vi "select_images.vi"(8 "error in (no error)":errorcluster, 9 "Select":bool, 10 "All":bool, 11 "dict of HIS IN":variant) -> (0 "error out":errorcluster, 3 "dict of HIS OUT":variant)   [LabVIEW 2015]
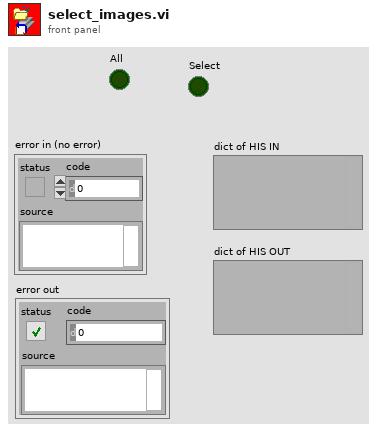
[diagram p1: front panel]
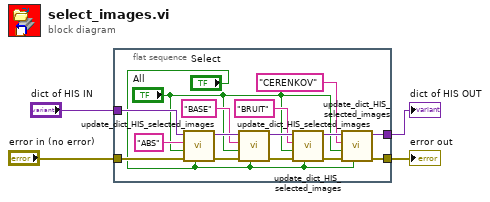
[diagram p0: block diagram]
diagram:
  n1 = flat-sequence {
    tunnel: "dict of HIS IN" -> [w20]
    tunnel: [w16] -> w3
    tunnel: "error in (no error)" -> [w15]
    tunnel: [w11] -> w1
    frame #0 {
      n2 = call "update_dict_HIS_selected_images.vi"("Select"="Select", "error in (no error)"=w15, "All"="All", "type"="ABS" ("name"), "dict of HIS IN"=w20) -> ("error out"=w14:errorcluster, "dict of HIS OUT"=w19:variant)  [unwired: 5 in]
      n3 = call "update_dict_HIS_selected_images.vi"("Select"="Select", "error in (no error)"=w14, "All"="All", "type"="BASE" ("name"), "dict of HIS IN"=w19) -> ("error out"=w13:errorcluster, "dict of HIS OUT"=w18:variant)  [unwired: 5 in]
      n4 = call "update_dict_HIS_selected_images.vi"("Select"="Select", "error in (no error)"=w13, "All"="All", "type"="BRUIT" ("name"), "dict of HIS IN"=w18) -> ("error out"=w12:errorcluster, "dict of HIS OUT"=w17:variant)  [unwired: 5 in]
      n5 = call "update_dict_HIS_selected_images.vi"("Select"="Select", "error in (no error)"=w12, "All"="All", "type"="CERENKOV" ("name"), "dict of HIS IN"=w17) -> ("error out"=w11:errorcluster, "dict of HIS OUT"=w16:variant)  [unwired: 5 in]
    }
  }
  "dict of HIS OUT" <- w3
  "error out" <- w1
